vi "XML - Read from XML.vi"(8 "error in (no error)":errorcluster, 11 "path to XML document":path caption="XML Path") -> (0 "error out":errorcluster, 2 "Rx Channel Info":T1[](array[typedef]) {"Data Type" items=["U8", "U16", "U32", "U64", "I8", "I16", "I32", "I64", "SGL", "DBL", "EXT"]}, 3 "Tx Channel Info":T1[](array[typedef]) {"Data Type" items=["U8", "U16", "U32", "U64", "I8", "I16", "I32", "I64", "SGL", "DBL", "EXT"]})   [LabVIEW 2016, in "UDP-Custom-Device System Explorer.lvlib"]
uses:
  UDP-Custom-Device System Explorer.lvlib
  Types/XML/XML - Channel.ctl
  <vilib>/xml/Load XML File.vi
  <vilib>/xml/Close Reference(Node).vi
  <vilib>/xml/NI_XML.lvlib
  <resource>/objmgr/DOMUserDefRef.rc
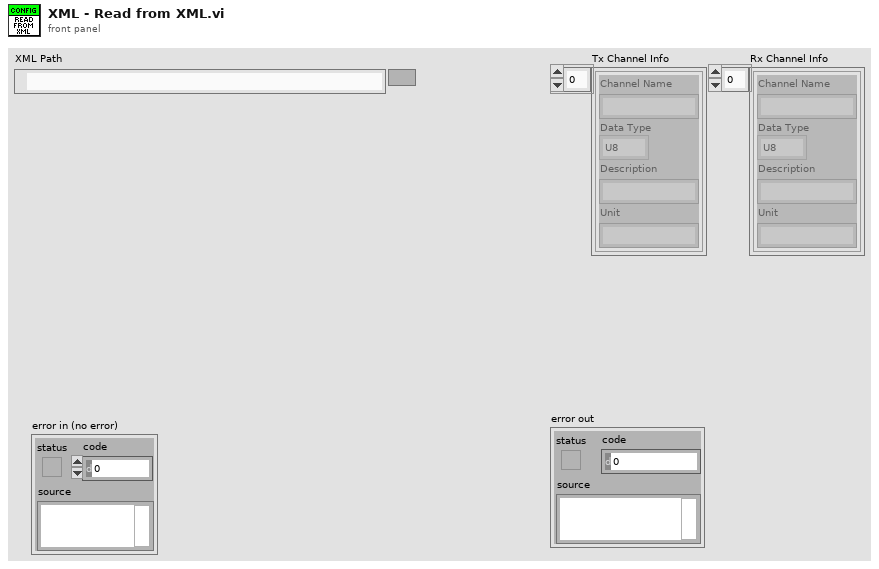
[diagram p1: front panel]
types:
  T1 = typedef "UDP-Custom-Device System Explorer.lvlib/XML - Channel.ctl" = cluster{"Channel Name":string, "Data Type":u16, "Description":string, "Unit":string}
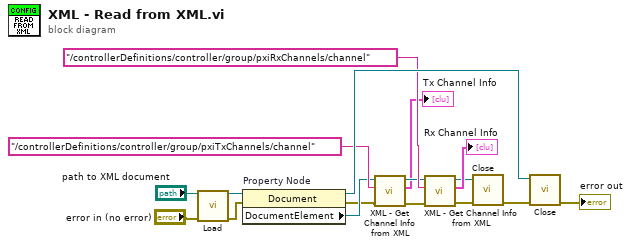
[diagram p0: block diagram]
diagram:
  n1 = call-poly <vilib>:"Load.vi"("path to XML document"="path to XML document", "error in (no error)"="error in (no error)") -> ("DOM document out"=w16:refnum<k20>, "error out"=w15:errorcluster)  [unwired: 11 in, 1 out]
  n2 = property on="Property Node" class="Document"(reference=w16, error in=w15) -> (reference out=w14:refnum<k20>, error out=w1:errorcluster, "DocumentElement"=w2:refnum<k20>)
  n3 = call "XML - Get Channel Info from XML.vi"("error in"=w1, "XPath expression"="/controllerDefinitions/controller/group/pxiTxChannels/channel", "Document Element Node in"=w2) -> ("error out"=w6:errorcluster, "Channel Info"=→"Tx Channel Info":T1[], "Document Element Node out"=w5:refnum<k20>)  [unwired: 6 in]
  n4 = call "XML - Get Channel Info from XML.vi"("error in"=w6, "XPath expression"="/controllerDefinitions/controller/group/pxiRxChannels/channel", "Document Element Node in"=w5) -> ("error out"=w7:errorcluster, "Channel Info"=→"Rx Channel Info":T1[], "Document Element Node out"=w8:refnum<k20>)  [unwired: 6 in]
  n5 = call-poly <vilib>:"Close.vi"("error in (no error)"=w7, "node"=w8) -> ("error out"=w13:errorcluster)  [unwired: 7 in]
  n6 = call-poly <vilib>:"Close.vi"("error in (no error)"=w13, "node"=w14) -> ("error out"=→"error out":errorcluster)  [unwired: 7 in]
